vi "FSM_new.vi"() -> ()   [LabVIEW 2016]
panel:
  out "note":string
  out "Waveform Graph 2":dbl[](graph)
  out "Select traing signal":i32
  out "Saved Target":dbl[][](array[numeric])
  out "Number of Signals":i32
  out "Signal Captured":dbl[][](array[numeric])
  in  "Signal Capture":bool
  out "Error_out":dbl[](array[numeric])
  out "Final Error":dbl
  out "Waveform Graph":dbl[](graph)
  in  "Inference":bool
  in  "Training":bool
  out "Enum":T1(ring)
  out "Weights_oX":dbl[][](array[numeric])
  out "Weights_hX":dbl[][](array[numeric])
  out "Outputs_oX":dbl[](array[numeric])
  out "Outputs_hX":dbl[](array[numeric])
  in  "Target 6":dbl
  in  "Target 5":dbl
  in  "Target 7":dbl
  in  "Target 8":dbl
  in  "Learning rate":dbl
  in  "Offset 2":dbl
  in  "Offset 1":dbl
  out "Random values generated":bool
  out "Training end":bool
  in  "Target 4":dbl
  in  "Target 3":dbl
  in  "Target 2":dbl
  in  "Target 1":dbl
  in  "Stop":bool
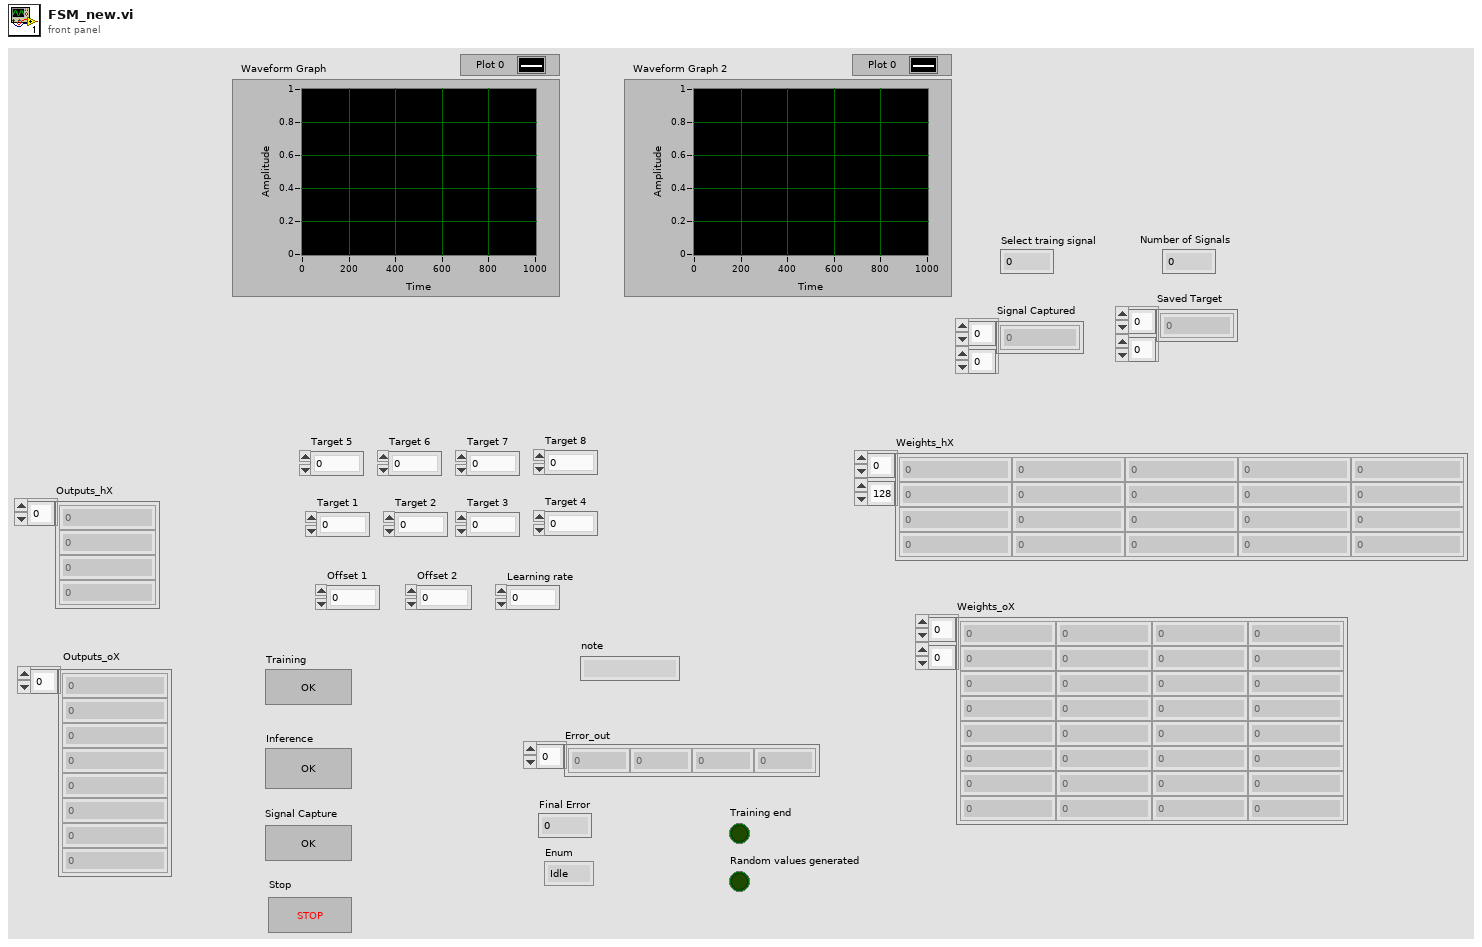
[diagram p1: front panel]
types:
  T1 = enum16{"Idle", "Generate weights", "Training mode", "Inference mode"}
  T2 = enum16{"Idle", "Generate weights", "Training mode", "Inference mode", "Signal Capture"}
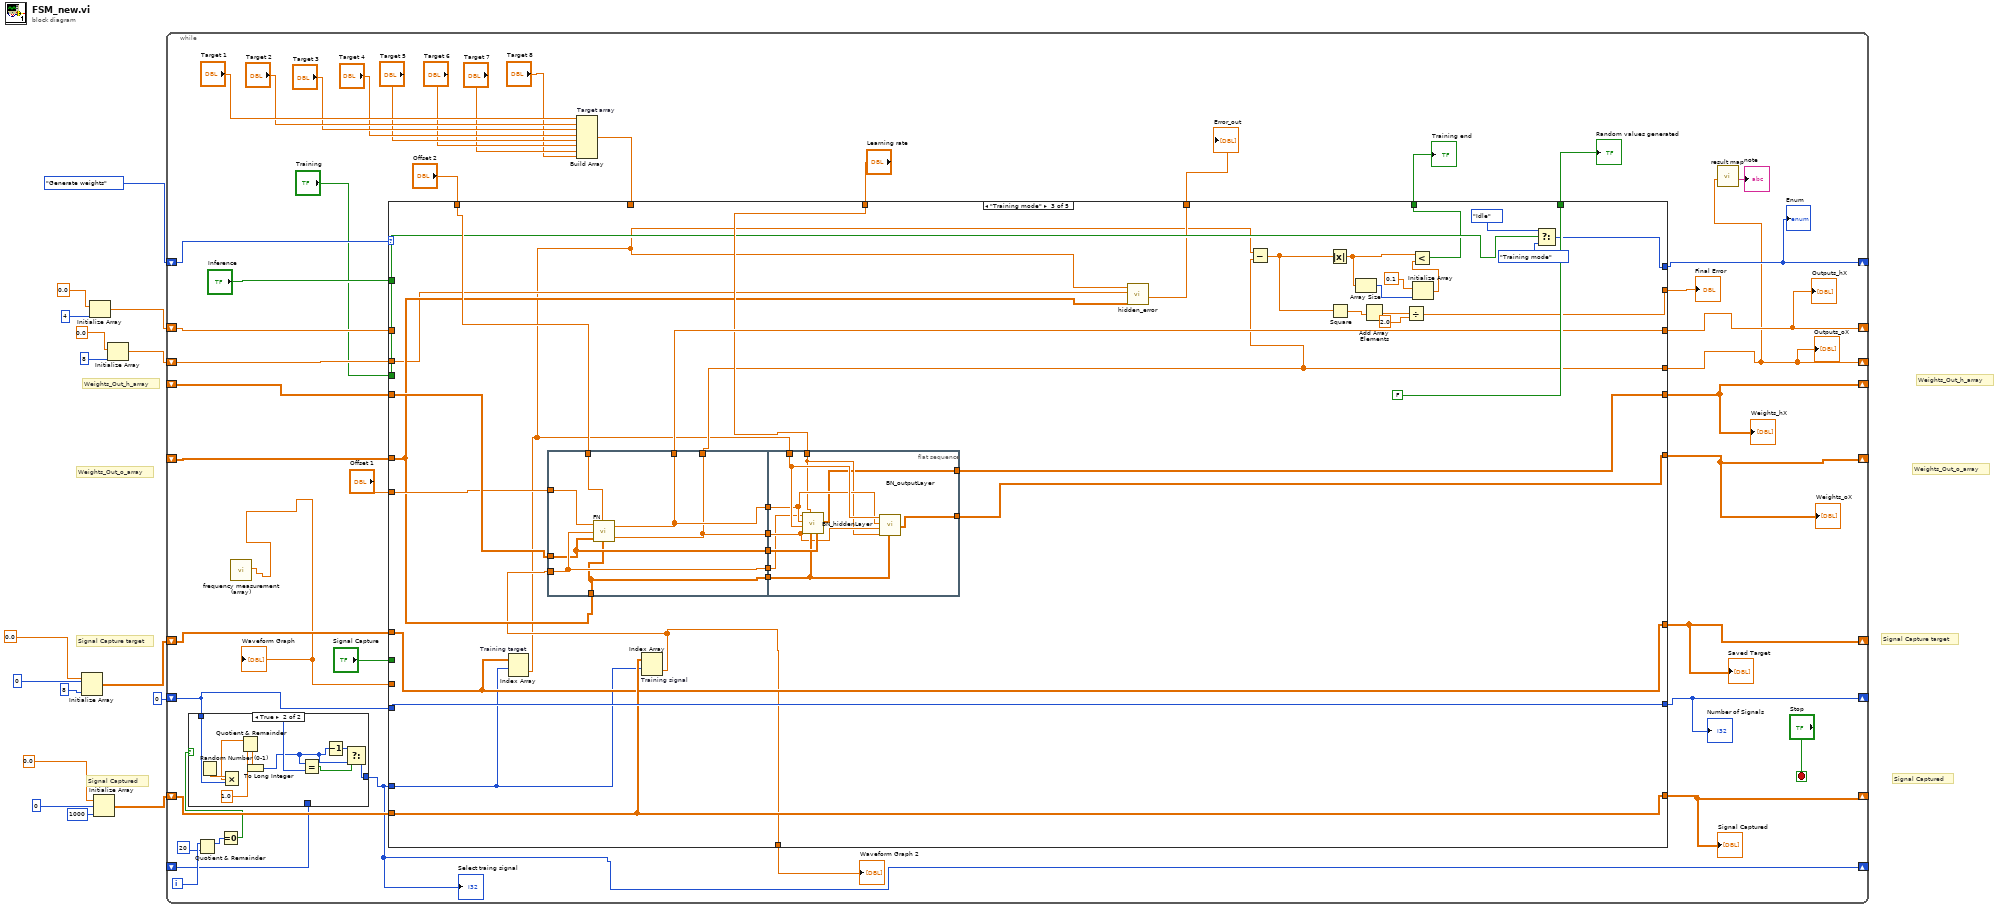
[diagram p0: block diagram]
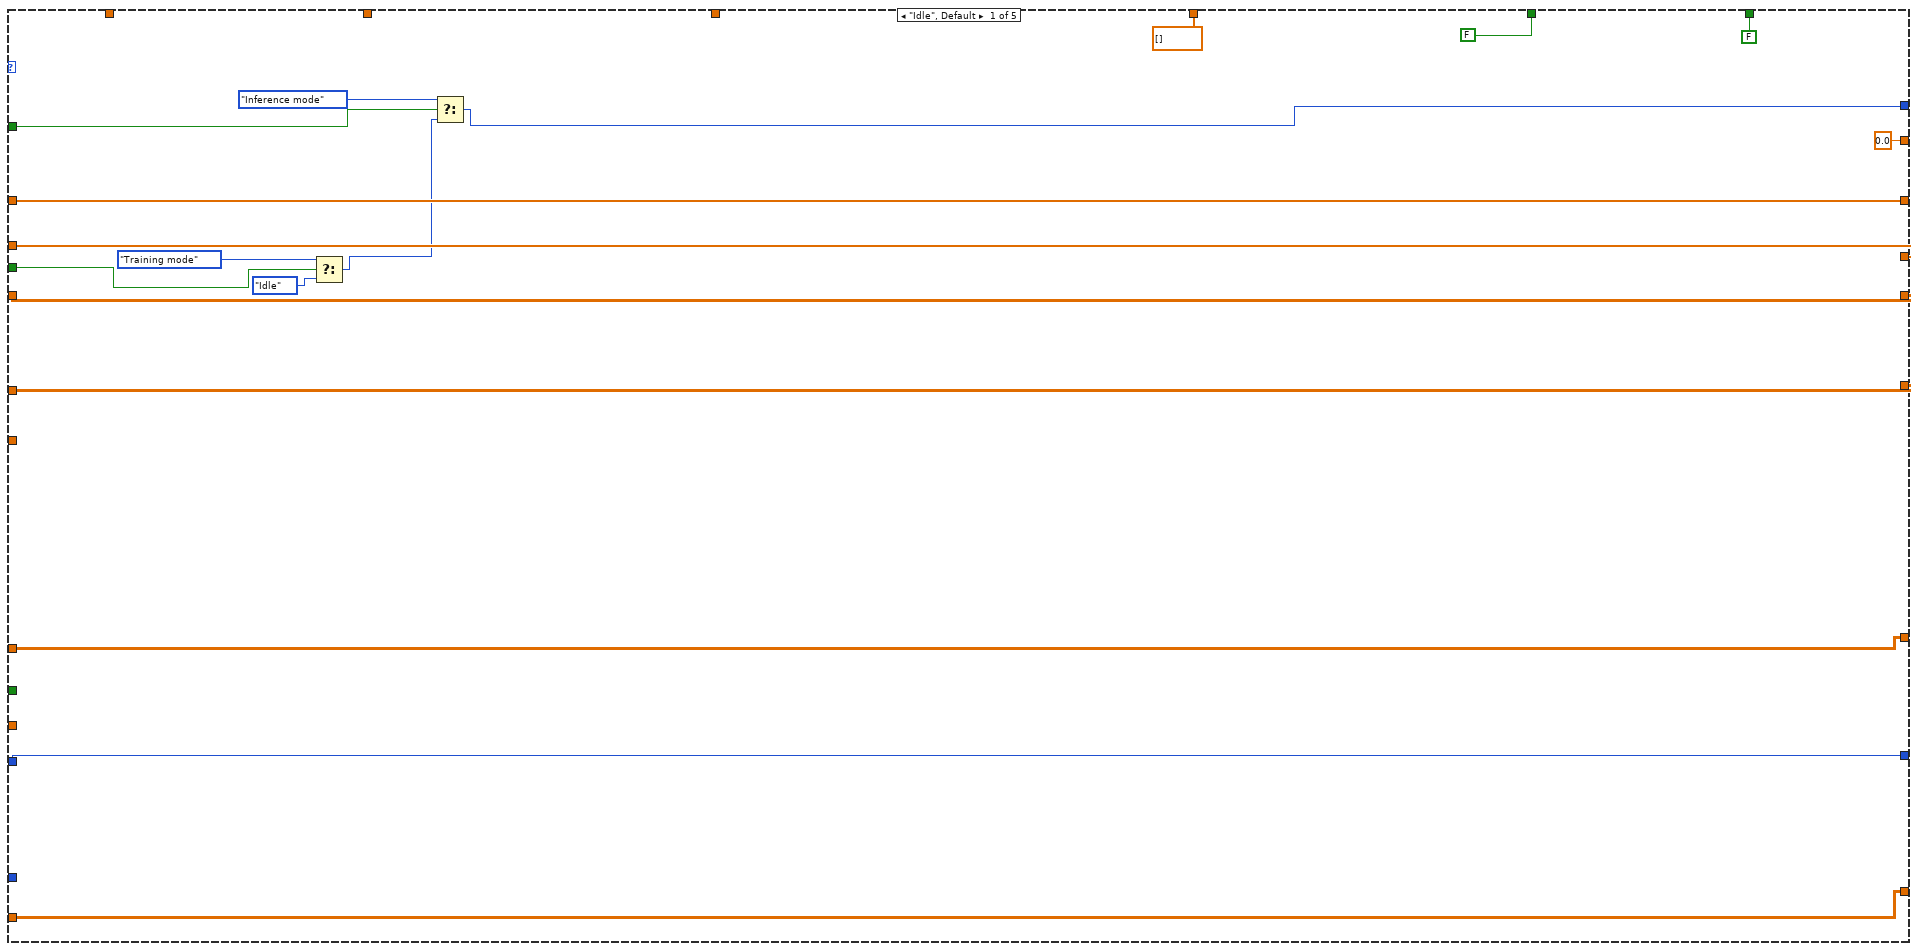
[diagram p3: hidden frame]
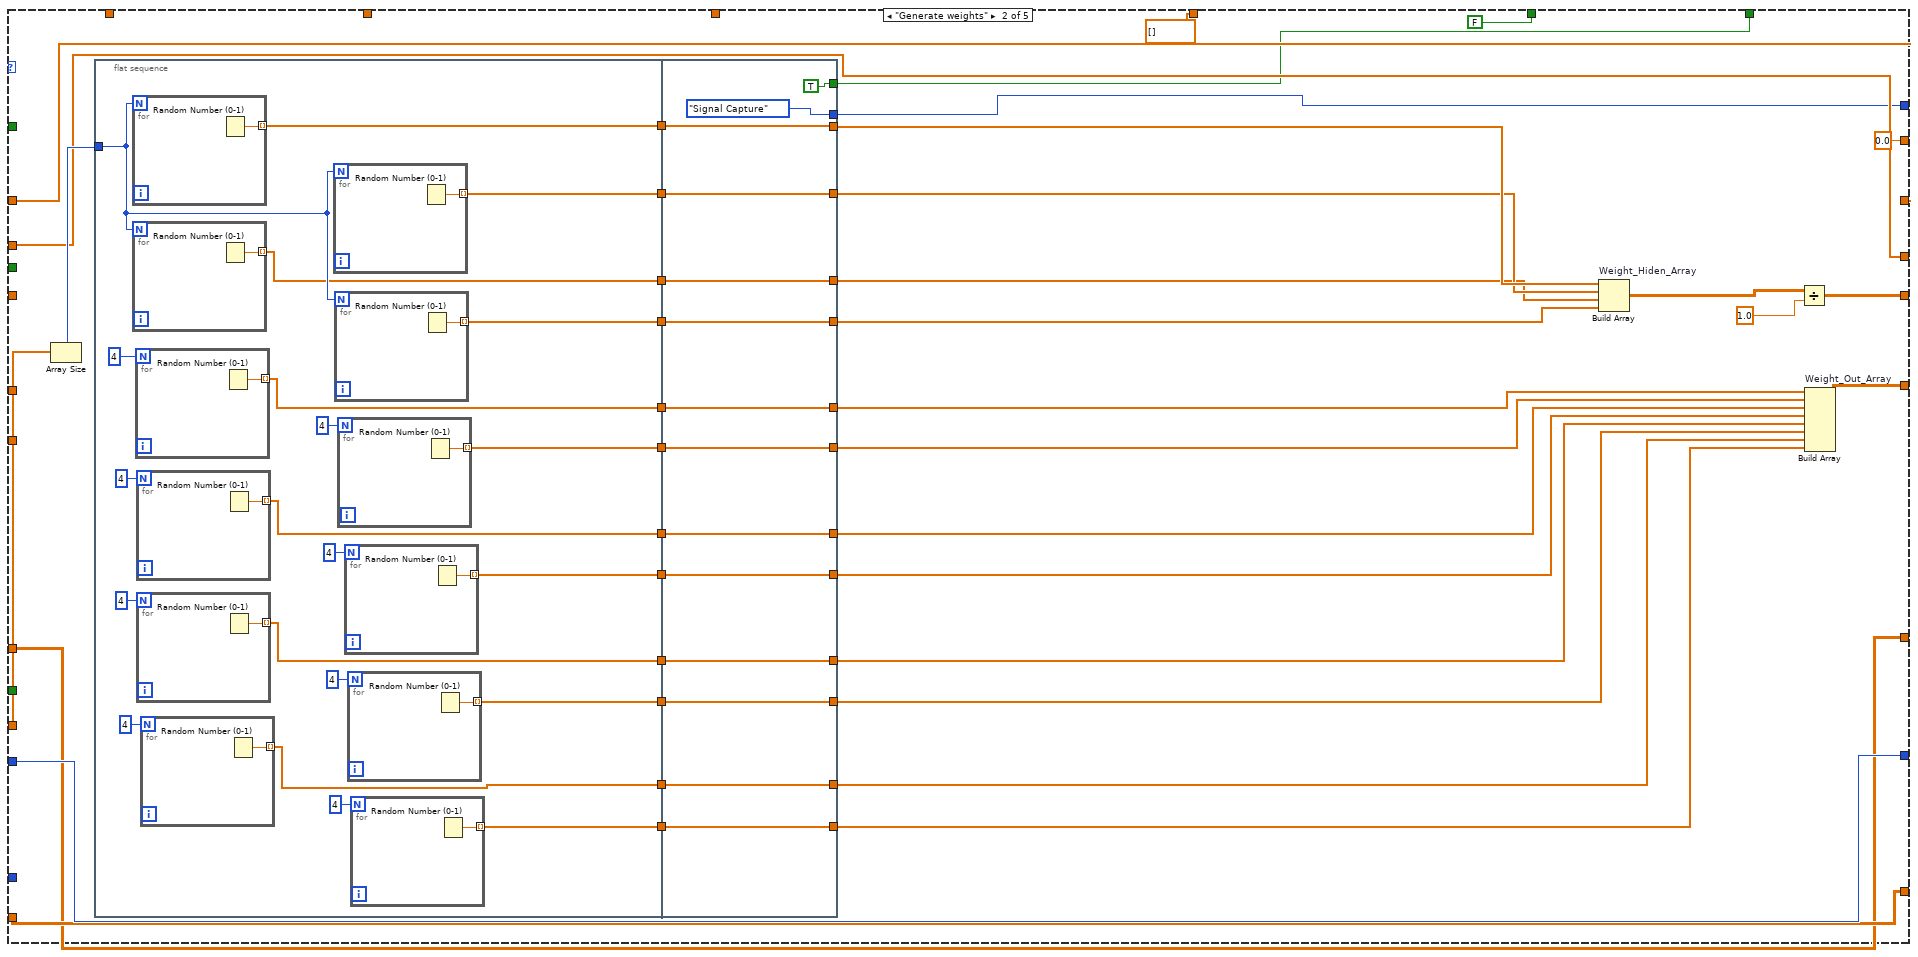
[diagram p4: hidden frame]
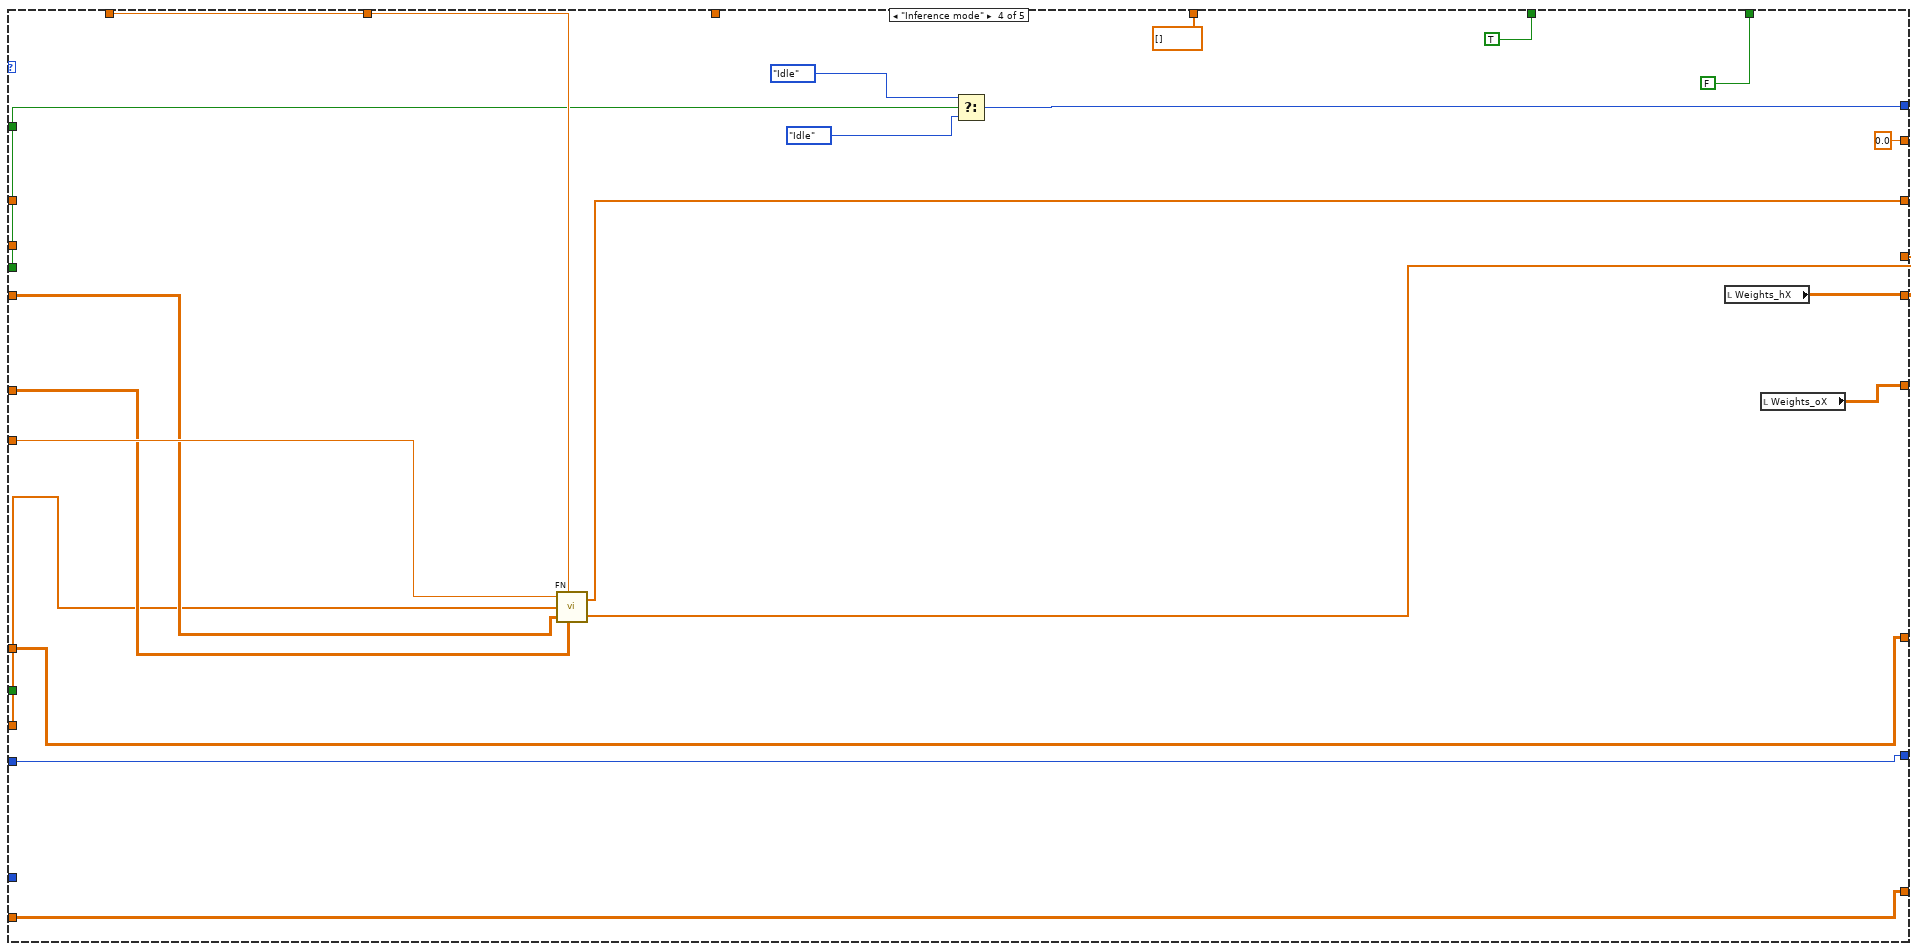
[diagram p5: hidden frame]
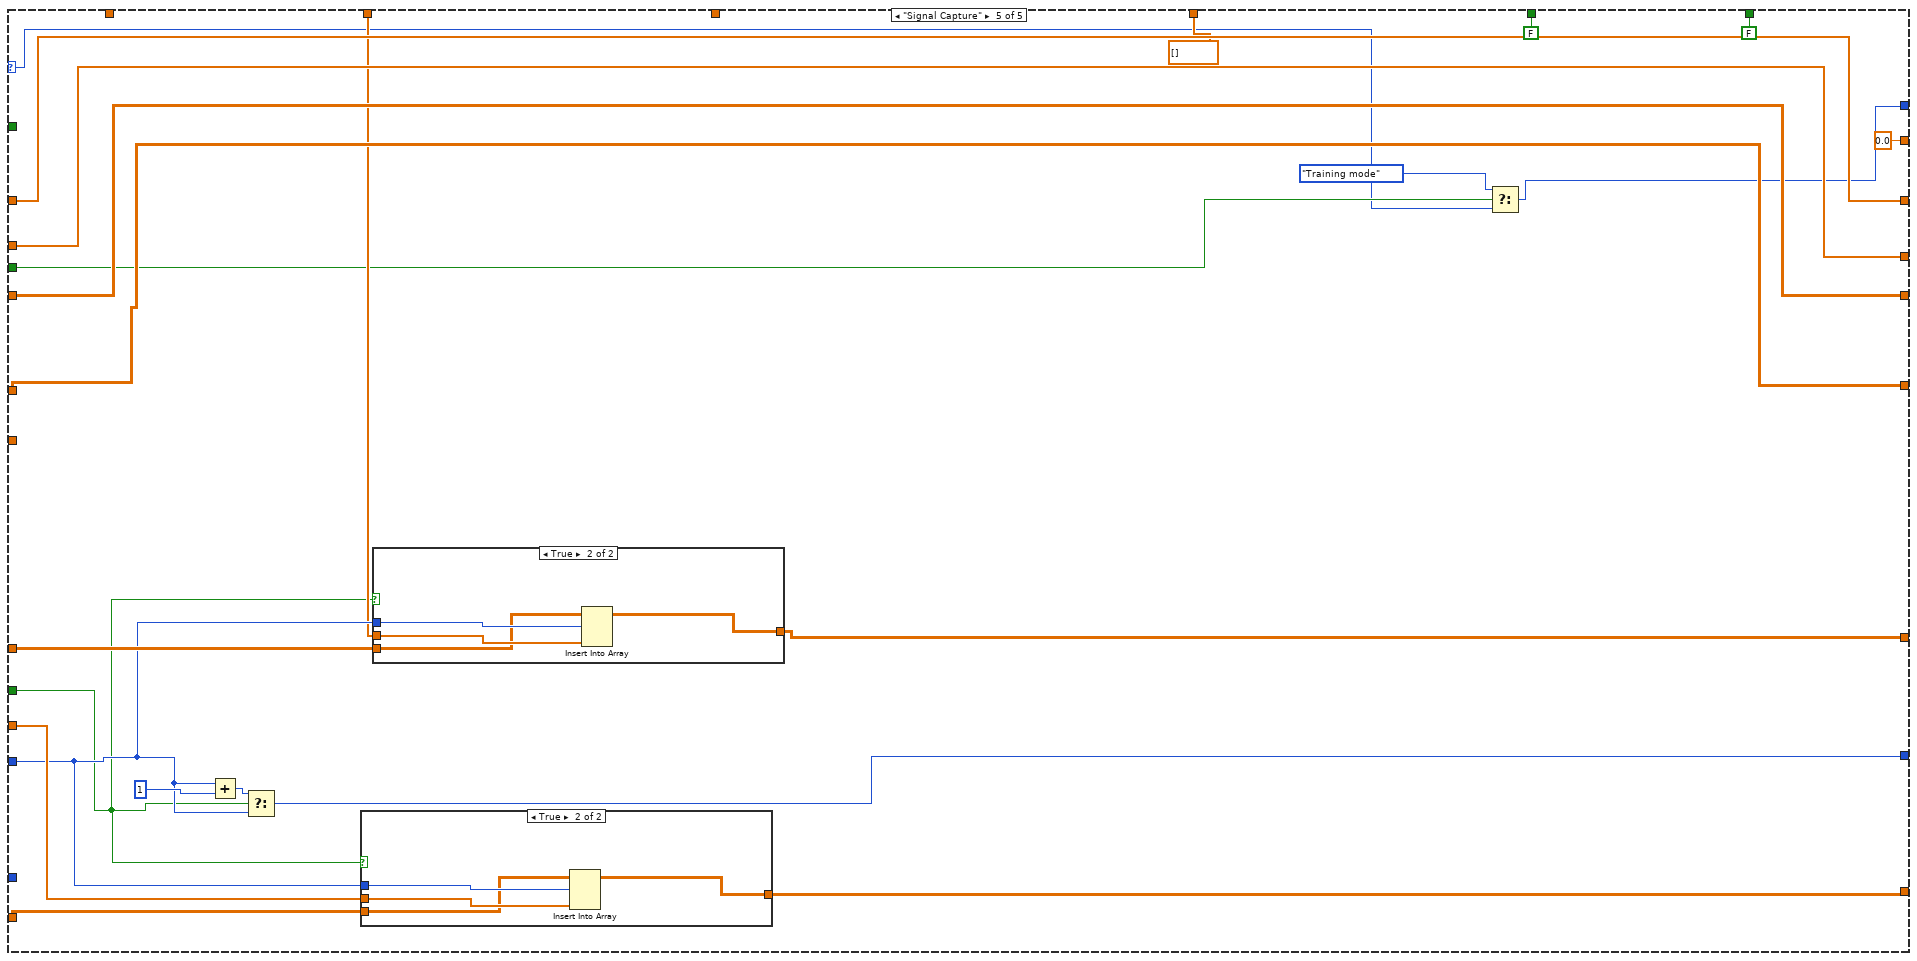
[diagram p6: hidden frame]
diagram:
  # "Signal Captured"
  # "Signal Capture target"
  # "Signal Captured"
  # "Signal Capture target"
  # "Weights_Out_o_array"
  # "Weights_Out_h_array"
  # "Weights_Out_o_array"
  # "Weights_Out_h_array"
  n1 = Initialize Array(0.0, 0, 8 ("dimension size")) -> (w1:dbl[][])
  n2 = Initialize Array(0.0, 4) -> (w15:dbl[])
  n3 = Initialize Array(0.0, 0, 1000 ("dimension size")) -> (w6:dbl[][])
  n4 = Initialize Array(0.0, 8) -> (w10:dbl[])
  n5 = while {
    shift-right: [w40] -> _
    shift-left: T2."Generate weights" -> [w57]
    shift-right: [w45] -> _
    shift-left: _ -> [w44]
    shift-right: [w46] -> _
    shift-left: _ -> [w43]
    shift-right: [w39] -> _
    shift-left: w15 -> [w42]
    shift-right: [w18] -> _
    shift-left: w10 -> [w41]
    shift-right: [w32] -> _
    shift-left: 0 -> [w25]
    shift-right: [w31] -> _
    shift-left: w6 -> [w30]
    shift-right: [w28] -> _
    shift-left: w1 -> [w29]
    shift-right: [w19] -> _
    shift-left: _ -> [w20]
    i -> [w24]
    stop <- "Stop" stop-if-true
    n6 = Quotient & Remainder(x=w24, y=20) -> (x-y*floor(x/y)=w22:i32)  [unwired: 1 out]
    n7 = Equal To 0?(x=w22) -> (x = 0?=w21:bool)
    n8 = case shown="True" w21 {
      tunnel: w25 -> [_ w67]
      tunnel: [w62 w63] -> w19
      tunnel: w20 -> [w62 _]
      frame False {
      }
      frame True {
        n9 = Random Number (0-1)() -> (number: 0 to 1=w71:dbl)
        n10 = Multiply(x=w71, y=w67) -> (x*y=w70:dbl)
        n11 = Quotient & Remainder(x=w70, y=1.0) -> (floor(x/y)=w68:dbl)  [unwired: 1 out]
        n12 = To Long Integer(number=w68) -> (32bit integer=w64:i32)
        n13 = Equal?(x=w64, y=w67) -> (x = y?=w66:bool)
        n14 = Decrement(x=w64) -> (x-1=w65:i32)
        n15 = Select(t=w65, s=w66, f=w64) -> (s? t:f=w63:i32)
      }
    }
    "Select traing signal" <- w19
    n16 = call "frequency measurement (array).vi"() -> ("real part of fft array"=w26:dbl[])  [unwired: 11 in]
    "Waveform Graph" <- w26
    n17 = Build Array "Target array"("Target 1", "Target 2", "Target 3", "Target 4", "Target 5", "Target 6", "Target 7", "Target 8") -> (w48:dbl[])
    n18 = case shown="\"Training mode\"" w57 {
      selector: w57 -> [_ _ _ _ w251]
      tunnel: [w77 w90 w199 w238 w253] -> w40
      tunnel: [FALSE w100 FALSE FALSE FALSE] -> w47
      tunnel: "Offset 1" -> [_ _ w211 w248 _]
      tunnel: "Offset 2" -> [_ _ w210 w249 _]
      tunnel: "Learning rate" -> [_ _ w208 _ _]
      tunnel: w48 -> [_ _ _ _ w256]
      tunnel: [w85 w103 w209 w247 w271] -> w39
      tunnel: [w84 w102 w202 w246 w270] -> w18
      tunnel: w26 -> [_ w101 _ w235 w261]
      tunnel: [w87 w97 w177 w244 w269] -> w45
      tunnel: [w86 w104 w194 w243 w268] -> w46
      tunnel: w44 -> [w87 _ w212 w242 w269]
      tunnel: w43 -> [w86 _ w186 w241 w268]
      tunnel: w42 -> [w85 w103 _ _ w271]
      tunnel: w41 -> [w84 w102 w185 _ w270]
      tunnel: "Training" -> [w82 _ w193 w237 w252]
      tunnel: [FALSE FALSE w192 TRUE FALSE] -> w38
      tunnel: "Inference" -> [w79 _ _ _ _]
      tunnel: [0.0 0.0 w187 0.0 0.0] -> w35
      tunnel: [dbl[] [] ("Error_out") dbl[] [] ("Error_out") w184 dbl[] [] ("Error_out") dbl[] [] ("Error_out")] -> w34
      tunnel: "Signal Capture" -> [_ _ _ _ w255]
      tunnel: [w73 w93 w183 w232 w262] -> w32
      tunnel: w25 -> [w73 w93 w183 w232 w257]
      tunnel: [w74 w92 w182 w231 w260] -> w31
      tunnel: w30 -> [w74 w92 w182 w231 w259]
      tunnel: w29 -> [w72 w91 w181 w230 w258]
      tunnel: [w72 w91 w181 w230 w254] -> w28
      tunnel: w19 -> [_ _ w178 _ _]
      tunnel: [_ _ w180 _ _] -> w27
      frame "Idle", Default {
        n19 = Select(t=T1."Training mode", s=w82, f=T1."Idle") -> (s? t:f=w78:T1)
        n20 = Select(t=T1."Inference mode", s=w79, f=w78) -> (s? t:f=w77:T1)
      }
      frame "Generate weights" {
        n21 = Array Size(array=w101) -> (size(s)=w129:i32)
        n22 = flat-sequence {
          tunnel: w129 -> [w150]
          tunnel: [w149] -> w128
          tunnel: [w148] -> w127
          tunnel: [w147] -> w126
          tunnel: [w146] -> w125
          tunnel: [w145] -> w124
          tunnel: [w144] -> w123
          tunnel: [w143] -> w122
          tunnel: [w142] -> w121
          tunnel: [w141] -> w120
          tunnel: [w140] -> w119
          tunnel: [w139] -> w118
          tunnel: [w138] -> w117
          tunnel: [TRUE] -> w100
          tunnel: w128 -> [w175]
          tunnel: [w175] -> w116
          tunnel: w127 -> [w174]
          tunnel: [w174] -> w114
          tunnel: w126 -> [w173]
          tunnel: [w173] -> w105
          tunnel: w125 -> [w172]
          tunnel: [w172] -> w107
          tunnel: w124 -> [w171]
          tunnel: [w171] -> w109
          tunnel: w123 -> [w170]
          tunnel: [w170] -> w111
          tunnel: w122 -> [w169]
          tunnel: [w169] -> w115
          tunnel: w121 -> [w168]
          tunnel: [w168] -> w113
          tunnel: w120 -> [w167]
          tunnel: [w167] -> w106
          tunnel: w119 -> [w166]
          tunnel: [w166] -> w108
          tunnel: [w165] -> w110
          tunnel: w118 -> [w165]
          tunnel: w117 -> [w164]
          tunnel: [w164] -> w112
          tunnel: [T2."Signal Capture"] -> w90
          frame #0 {
            n23 = for {
              N: w150 -> [_]
              tunnel: [w162] -> w149 mode=indexing
              n24 = Random Number (0-1)() -> (number: 0 to 1=w162:dbl)
            }
            n25 = for {
              N: w150 -> [_]
              tunnel: [w161] -> w148 mode=indexing
              n26 = Random Number (0-1)() -> (number: 0 to 1=w161:dbl)
            }
            n27 = for {
              N: 4 -> [_]
              tunnel: [w160] -> w147 mode=indexing
              n28 = Random Number (0-1)() -> (number: 0 to 1=w160:dbl)
            }
            n29 = for {
              N: 4 -> [_]
              tunnel: [w156] -> w146 mode=indexing
              n30 = Random Number (0-1)() -> (number: 0 to 1=w156:dbl)
            }
            n31 = for {
              N: 4 -> [_]
              tunnel: [w158] -> w145 mode=indexing
              n32 = Random Number (0-1)() -> (number: 0 to 1=w158:dbl)
            }
            n33 = for {
              N: 4 -> [_]
              tunnel: [w159] -> w144 mode=indexing
              n34 = Random Number (0-1)() -> (number: 0 to 1=w159:dbl)
            }
            n35 = for {
              N: w150 -> [_]
              tunnel: [w157] -> w143 mode=indexing
              n36 = Random Number (0-1)() -> (number: 0 to 1=w157:dbl)
            }
            n37 = for {
              N: w150 -> [_]
              tunnel: [w155] -> w142 mode=indexing
              n38 = Random Number (0-1)() -> (number: 0 to 1=w155:dbl)
            }
            n39 = for {
              N: 4 -> [_]
              tunnel: [w154] -> w141 mode=indexing
              n40 = Random Number (0-1)() -> (number: 0 to 1=w154:dbl)
            }
            n41 = for {
              N: 4 -> [_]
              tunnel: [w153] -> w140 mode=indexing
              n42 = Random Number (0-1)() -> (number: 0 to 1=w153:dbl)
            }
            n43 = for {
              N: 4 -> [_]
              tunnel: [w152] -> w139 mode=indexing
              n44 = Random Number (0-1)() -> (number: 0 to 1=w152:dbl)
            }
            n45 = for {
              N: 4 -> [_]
              tunnel: [w151] -> w138 mode=indexing
              n46 = Random Number (0-1)() -> (number: 0 to 1=w151:dbl)
            }
          }
          frame #1 {
          }
        }
        n47 = Build Array "Weight_Hiden_Array"(w116, w115, w114, w113) -> (w98:dbl[][])
        n48 = Divide(x=w98, y=1.0) -> (x/y=w97:dbl[][])
        n49 = Build Array "Weight_Out_Array"(w105, w106, w107, w108, w109, w110, w111, w112) -> (w104:dbl[][])
      }
      frame "Training mode" {
        n50 = Index Array "Training target"(array=w181, index (row)=w178) -> (element=w179:dbl[])  [unwired: 1 in]
        n51 = flat-sequence {
          tunnel: w180 -> [w218]
          tunnel: w212 -> [w216]
          tunnel: w186 -> [w215]
          tunnel: w211 -> [w220]
          tunnel: w210 -> [w219]
          tunnel: [w217] -> w209
          tunnel: [w214] -> w202
          tunnel: [w218] -> w207
          tunnel: [w217] -> w206
          tunnel: [w214] -> w205
          tunnel: [w216] -> w204
          tunnel: [w215] -> w203
          tunnel: w208 -> [w222]
          tunnel: [w229] -> w194
          tunnel: w207 -> [w223]
          tunnel: w206 -> [w224]
          tunnel: w179 -> [w225]
          tunnel: w205 -> [w226]
          tunnel: w204 -> [w228]
          tunnel: w203 -> [w227]
          tunnel: [w221] -> w177
          frame #0 {
            n52 = call "FN.vi"("Offset_h"=w220, "Offset_out"=w219, "Inputs"=w218, "Weights_h"=w216, "Weights_out"=w215) -> ("Outputs_hx"=w217:dbl[], "Outputs_out"=w214:dbl[])
          }
          frame #1 {
            n53 = call "BN_hiddenLayer.vi"("Weights_hX_IN"=w228, "Weights_outX(before being updated)"=w227, "Learning rate"=w222, "Out_outX"=w226, "Target_outX"=w225, "Out_hx"=w224, "Inputs"=w223) -> ("Weights_hX_OUT"=w221:dbl[][])  [unwired: 3 in]
            n54 = call "BN_outputLayer.vi"("Target_outX"=w225, "Out_hx"=w224, "Out_outX"=w226, "Learning rate"=w222, "Weights_outX_IN"=w227) -> ("Weights_outX_OUT"=w229:dbl[][])
          }
        }
        n55 = Index Array "Training signal"(array=w182, index (row)=w178) -> (element=w180:dbl[])  [unwired: 1 in]
        n56 = call "hidden_error.vi"("Weight"=w186, "Output"=w185, "Target"=w179) -> ("Error_out"=w184:dbl[])  [unwired: 8 in]
        n57 = Subtract(x=w179, y=w202) -> (x-y=w191:dbl[])
        n58 = Absolute Value(x=w191) -> (abs(x)=w197:dbl[])
        n59 = Square(x=w191) -> (x^2=w190:dbl[])
        n60 = Array Size(array=w197) -> (size(s)=w196:i32)
        n61 = Add Array Elements(numeric array=w190) -> (sum=w189:dbl)
        n62 = Divide(x=w189, y=2.0) -> (x/y=w187:dbl)
        n63 = Initialize Array(0.1 ("y"), w196) -> (w195:dbl[])
        n64 = Less?(x=w197, y=w195) -> (x < y?=w192:bool)
        n65 = Select(t=T1."Idle", s=w193, f=T1."Training mode") -> (s? t:f=w199:T1)
      }
      frame "Inference mode" {
        n66 = call "FN.vi"("Offset_h"=w248, "Offset_out"=w249, "Inputs"=w235, "Weights_h"=w242, "Weights_out"=w241) -> ("Outputs_hx"=w247:dbl[], "Outputs_out"=w246:dbl[])
        n67 = Select(t=T1."Idle", s=w237, f=T1."Idle") -> (s? t:f=w238:T1)
        n68 = local read "Weights_hX"() -> (w244:dbl[][])
        n69 = local read "Weights_oX"() -> (w243:dbl[][])
      }
      frame "Signal Capture" {
        n70 = Add(x=w257, y=1) -> (x+y=w264:i32)
        n71 = Select(t=w264, s=w255, f=w257) -> (s? t:f=w262:i32)
        n72 = case shown="True" w255 {
          tunnel: w257 -> [_ w282]
          tunnel: w261 -> [_ w281]
          tunnel: [w278 w280] -> w260
          tunnel: w259 -> [w278 w279]
          frame False {
          }
          frame True {
            n73 = Insert Into Array(array=w279, index (row)=w282, new element=w281) -> (w280:dbl[][])  [unwired: 1 in]
          }
        }
        n74 = case shown="True" w255 {
          tunnel: w257 -> [_ w277]
          tunnel: w256 -> [_ w276]
          tunnel: [w273 w275] -> w254
          tunnel: w258 -> [w273 w274]
          frame False {
          }
          frame True {
            n75 = Insert Into Array(array=w274, index (row)=w277, new element=w276) -> (w275:dbl[][])  [unwired: 1 in]
          }
        }
        n76 = Select(t=T2."Training mode", s=w252, f=w251) -> (s? t:f=w253:T2)
      }
    }
    "Weights_hX" <- w45
    "Weights_oX" <- w46
    "Random values generated" <- w47
    "Enum" <- w40
    "Outputs_hX" <- w39
    "Outputs_oX" <- w18
    "Training end" <- w38
    "Final Error" <- w35
    "Error_out" <- w34
    "Number of Signals" <- w32
    "Signal Captured" <- w31
    "Saved Target" <- w28
    "Waveform Graph 2" <- w27
    n77 = call "result map.vi"("output"=w18) -> ("note"=→"note":string)  [unwired: 10 in]
  }
